vi "libssh2_session_init_ex.vi"(7 "abstract":u64, 8 "error in (no error)":errorcluster, 9 "myrealloc":u64, 10 "myfree":u64, 11 "myalloc":u64) -> (0 "error out":errorcluster, 3 "session":T1)   [LabVIEW 2013, in "libssh2.lvlib"]
doc: "Initializes a <B>session</B> object."
uses:
  libssh2.lvlib
  Session Refnum.ctl
  libssh2.dll
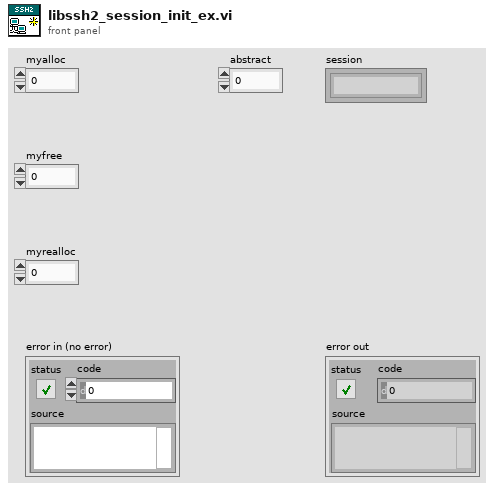
[diagram p1: front panel]
types:
  T1 = typedef "libssh2.lvlib/Session Refnum.ctl" = refnum<k1>
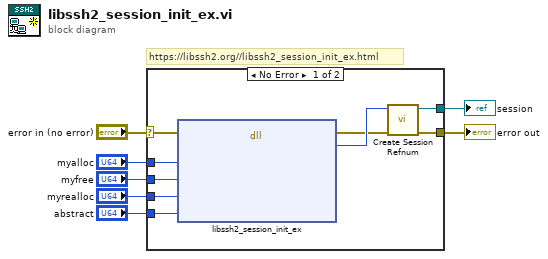
[diagram p0: block diagram]
diagram:
  # "https://libssh2.org//libssh2_session_init_ex.html"
  n1 = case shown="No Error" "error in (no error)" {
    selector: "error in (no error)" -> [w8 w17]
    tunnel: "myalloc" -> [w16 _]
    tunnel: "myfree" -> [w15 _]
    tunnel: "myrealloc" -> [w14 _]
    tunnel: "abstract" -> [w13 _]
    tunnel: [w11 _] -> w3
    tunnel: [w9 w17] -> w2
    frame No Error {
      n2 = dll-call lib="C:/Users/pasca/source/repos/libssh2-labview/libssh2**.*" fn="libssh2_session_init_ex"(error in=w8, "myalloc"=w16, "myfree"=w15, "myrealloc"=w14, "abstract"=w13) -> (error out=w10:errorcluster, "return value"=w12:u64)  [unwired: 6 in, 1 out]
      n3 = call "Create Session Refnum.vi"("error in (no error)"=w10, "LIBSSH2_SESSION*"=w12) -> ("error out"=w9:errorcluster, "session"=w11:T1)  [unwired: 8 in]
    }
    frame Error {
    }
  }
  "session" <- w3
  "error out" <- w2
